vi "SrsQcm200FandR_MODIFIED.vi"(0 "VISA in":refnum<visa-resource-name>="GPIB0::3::INSTR", 1 "Reference time in":u32, 11 "error in (no error)":errorcluster) -> (4 "VISA out":refnum<visa-resource-name>, 6 "Frequency out":dbl format="%.6f", 8 "timestamp out":dbl format="%.2f", 10 "Resistance out":dbl format="%.6f", 13 "F vs T out":T2 {"Frequency out" format="%.2f"; "timestamp out" format="%.2f"}, 14 "R vs T out":T1 {"Resistance out" format="%.2f"; "timestamp out" format="%.2f"}, 15 "error out":errorcluster)   [LabVIEW 2014]
doc: "This VI returns the QCM200 frequency and resistance values together.\n\nCopyright 2004 Stanford Research Systems"
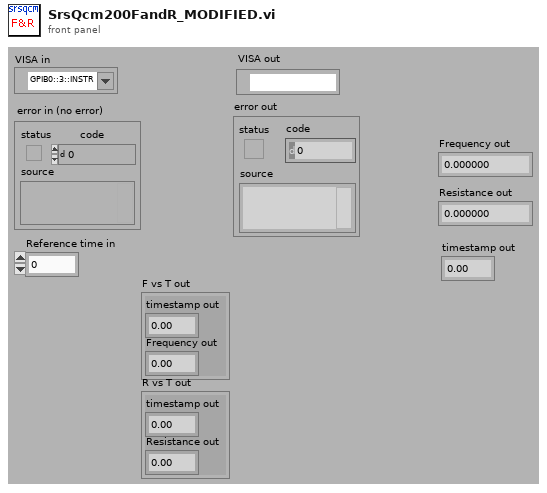
[diagram p1: front panel]
types:
  T1 = cluster{"timestamp out":dbl, "Resistance out":dbl}
  T2 = cluster{"timestamp out":dbl, "Frequency out":dbl}
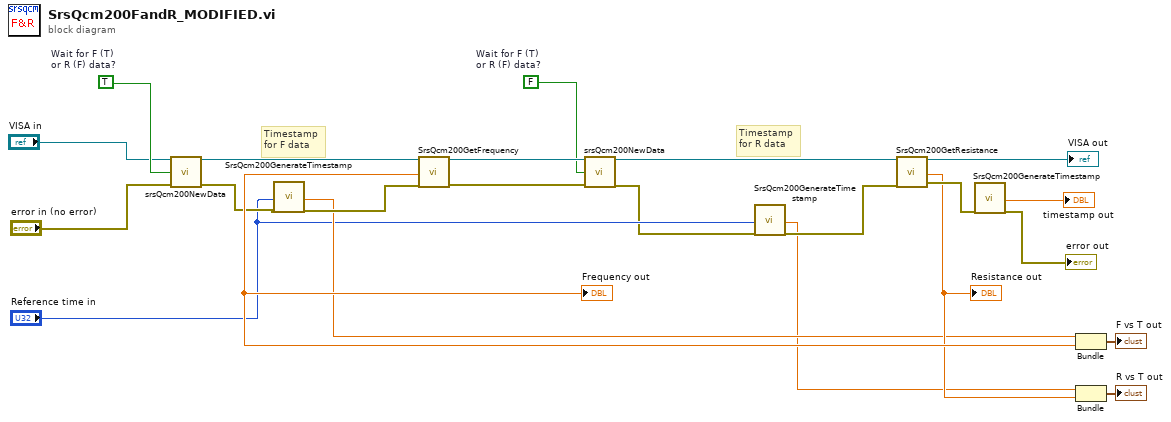
[diagram p0: block diagram]
diagram:
  w20 = FALSE  # Wait for F (T) or R (F) data?
  w19 = TRUE  # Wait for F (T) or R (F) data?
  # "Timestamp\nfor R data"
  # "Timestamp\nfor F data"
  n1 = call "srsQcm200NewData.vi"("VISA in"="VISA in", "Wait for F (T)\nor R (F) data?"=w19, "error in (no error)"="error in (no error)") -> ("VISA out"=w23:refnum<visa-resource-name>, "error out"=w8:errorcluster)  [unwired: 11 in]
  n2 = call "SrsQcm200GenerateTimestamp.vi"("Reference time in"="Reference time in", "Error In"=w8) -> ("timestamp out"=w5:dbl, "error out"=w7:errorcluster)  [unwired: 16 in]
  n3 = call "SrsQcm200GetFrequency.vi"("VISA in"=w23, "error in (no error)"=w7) -> ("VISA out"=w21:refnum<visa-resource-name>, "Frequency out"=w12:dbl, "error out"=w22:errorcluster)  [unwired: 15 in]
  "Frequency out" <- w12
  n4 = call "srsQcm200NewData.vi"("VISA in"=w21, "Wait for F (T)\nor R (F) data?"=w20, "error in (no error)"=w22) -> ("VISA out"=w16:refnum<visa-resource-name>, "error out"=w3:errorcluster)  [unwired: 11 in]
  n5 = call "SrsQcm200GenerateTimestamp.vi"("Reference time in"="Reference time in", "Error In"=w3) -> ("timestamp out"=w1:dbl, "error out"=w2:errorcluster)  [unwired: 16 in]
  n6 = call "SrsQcm200GetResistance.vi"("VISA in"=w16, "error in (no error)"=w2) -> ("VISA out"=→"VISA out":refnum<visa-resource-name>, "Resistance out"=w10:dbl, "error out"=w14:errorcluster)  [unwired: 15 in]
  "Resistance out" <- w10
  n7 = call "SrsQcm200GenerateTimestamp.vi"("Error In"=w14) -> ("timestamp out"=→"timestamp out":dbl, "error out"=→"error out":errorcluster)  [unwired: 17 in]
  n8 = Bundle("timestamp out"=w5, "Frequency out"=w12) -> (→"F vs T out":T2)  [unwired: 1 in]
  n9 = Bundle("timestamp out"=w1, "Resistance out"=w10) -> (→"R vs T out":T1)  [unwired: 1 in]
